vi "mean11.vi"(2 "Y":i16[](array[numeric])) -> (6 "mean":sgl, 7 "dY":i16, 8 "std":sgl)   [LabVIEW 2010]
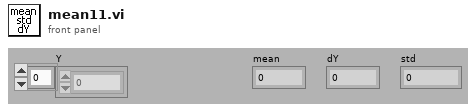
[diagram p1: front panel]
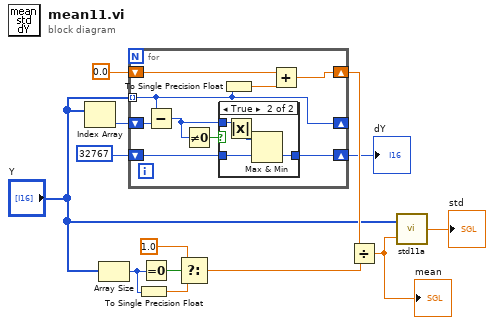
[diagram p0: block diagram]
diagram:
  n1 = Index Array(array="Y") -> (element=w4:i16)  [unwired: 1 in]
  n2 = Array Size(array="Y") -> (size(s)=w8:i32)
  n3 = for {
    shift-right: [w17] -> _
    shift-left: w4 -> [w22]
    tunnel: "Y" -> [w17] mode=indexing
    shift-right: [w19] -> w5
    shift-left: i16 32767 ("max(x,y)") -> [w18]
    shift-right: [w15] -> w13
    shift-left: sgl 0.0 -> [w14]
    n4 = Subtract(x=w17, y=w22) -> (x-y=w21:i16)
    n5 = Not Equal To 0?(x=w21) -> (x != 0?=w20:bool)
    n6 = case shown="True" w20 {
      tunnel: w21 -> [_ w26]
      tunnel: [w23 w25] -> w19
      tunnel: w18 -> [w23 w24]
      frame False {
      }
      frame True {
        n7 = Absolute Value(x=w26) -> (abs(x)=w27:i16)
        n8 = Max & Min(x=w27, y=w24) -> (min(x,y)=w25:i16)  [unwired: 1 out]
      }
    }
    n9 = To Single Precision Float(number=w17) -> (single precision float=w16:sgl)
    n10 = Add(x=w14, y=w16) -> (x+y=w15:sgl)
  }
  "dY" <- w5
  n11 = To Single Precision Float(number=w8) -> (single precision float=w10:sgl)
  n12 = Equal To 0?(x=w8) -> (x = 0?=w9:bool)
  n13 = Select(t=sgl 1.0, s=w9, f=w10) -> (s? t:f=w6:sgl)
  n14 = Divide(x=w13, y=w6) -> (x/y=w7:sgl)
  "mean" <- w7
  n15 = call "std11a.vi"("mean"=w7, "Y"="Y") -> ("std"=→"std":sgl)
